vi "RDV-addDataToGraph.vi"(8 "error in (no error)":errorcluster, 11 "RDV-Reflection_Data_viewer in":refnum<class "RDV-Reflection_Data_viewer.lvclass">) -> (0 "error out":errorcluster, 3 "RDV-Reflection_Data_viewer out":refnum<class "RDV-Reflection_Data_viewer.lvclass">)   [LabVIEW 2020, in "RDV-Reflection_Data_viewer.lvclass"]
uses:
  RDV-Reflection_Data_viewer.lvclass
  RDV-Reflection_Data_viewer.lvclass/RDV-Reflection_Data_viewer.ctl
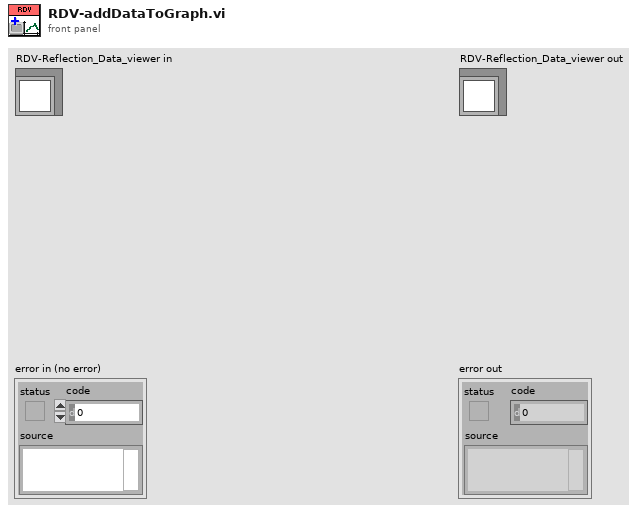
[diagram p1: front panel]
types:
  T1 = typedef "RDV-Reflection_Data_viewer.lvclass/RDV-XY_GRAPH_REFS.ctl" = cluster{"Reflection Real":refnum<vi>, "Reflection Imag":refnum<vi>, "Permittivity Real":refnum<vi>, "Permittivity Imag":refnum<vi>}
  T2 = cluster{"Frequency":dbl[], "Reflection'":dbl[]}[]
  T3 = cluster{"Frequency":dbl[], "Reflection'":dbl[]}[][]
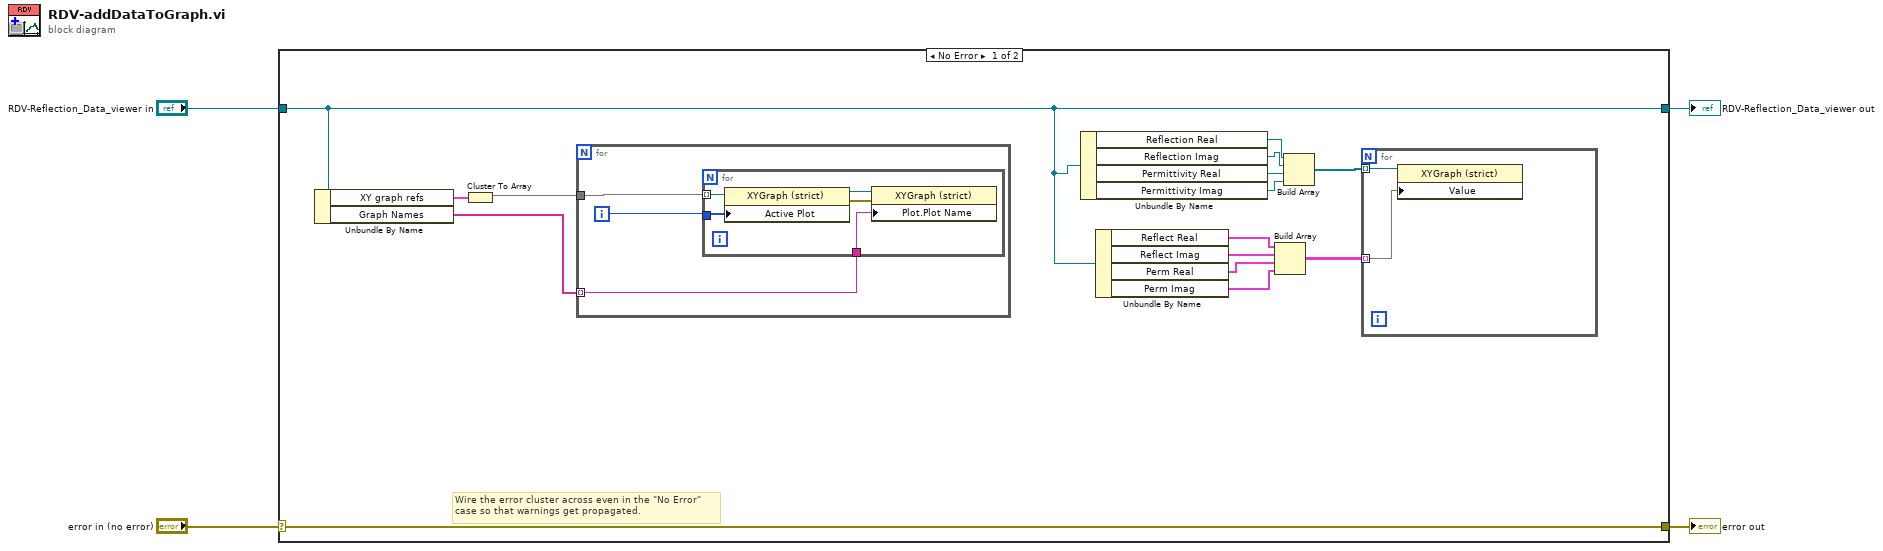
[diagram p0: block diagram]
diagram:
  n1 = case shown="No Error" "error in (no error)" {
    selector: "error in (no error)" -> [w19 w31]
    tunnel: [w19 w31] -> w3
    tunnel: [w11 w30] -> w1
    tunnel: "RDV-Reflection_Data_viewer in" -> [w11 w30]
    frame No Error {
      # "Wire the error cluster across even in the \"No Error\"\ncase so that warnings get propagated."
      n2 = Unbundle By Name(w11) -> ("XY graph refs"=w17:T1, "Graph Names"=w18:string[])
      n3 = Cluster To Array(cluster=w17) -> (array=w12:refnum<vi>[])
      n4 = for {
        tunnel: w12 -> [w21]
        tunnel: w18 -> [w20] mode=indexing
        i -> [w22]
        n5 = for {
          tunnel: w22 -> [w27]
          tunnel: w20 -> [w26]
          tunnel: w21 -> [w25] mode=indexing
          n6 = property on="Property Node" class="XYGraph (strict)"(reference=w25, "Active Plot"=w27) -> (reference out=w24:refnum<vi>, error out=w23:errorcluster)  [unwired: 1 in]
          n7 = property on="Property Node" class="XYGraph (strict)"(reference=w24, error in=w23, "Plot.Plot Name"=w26) -> ()  [unwired: 2 out]
        }
      }
      n8 = Unbundle By Name(w11) -> ("Reflection Real"=w10:refnum<vi>, "Reflection Imag"=w9:refnum<vi>, "Permittivity Real"=w8:refnum<vi>, "Permittivity Imag"=w7:refnum<vi>)
      n9 = Unbundle By Name(w11) -> ("Reflect Real"=w16:T2, "Reflect Imag"=w15:T2, "Perm Real"=w14:T2, "Perm Imag"=w13:T2)
      n10 = Build Array(w16, w15, w14, w13) -> (w5:T3)
      n11 = Build Array(w10, w9, w8, w7) -> (w6:refnum<vi>[])
      n12 = for {
        tunnel: w6 -> [w29] mode=indexing
        tunnel: w5 -> [w28] mode=indexing
        n13 = property on="Property Node" class="XYGraph (strict)"(reference=w29, "Value"=w28) -> ()  [unwired: 1 in, 2 out]
      }
    }
    frame Error {
    }
  }
  "error out" <- w3
  "RDV-Reflection_Data_viewer out" <- w1
